vi "Nema GPGGA string to UTM and time.vi"(9 "Grennich Offset":dbl=-8.0, 10 "Antenna offset":dbl max=0.0, 11 "String In (NEAMA GGA)":string="$GPGGA,152703.40,3814.751152,N,12130.720799,W,2,07,1.1,-5.47,M,-23.44,M,3.2,0211\n*5E") -> (0 "date/time string":string, 1 "Elevation":dbl format="%#_8g", 2 "Easting (M)":dbl format="%#.10g", 3 "Northing (M)":dbl format="%#.10g", 4 "Zone (string)":string)   [LabVIEW 2011]
uses:
  <vilib>/Utility/miscctls.llb/LVDateTimeRec.ctl
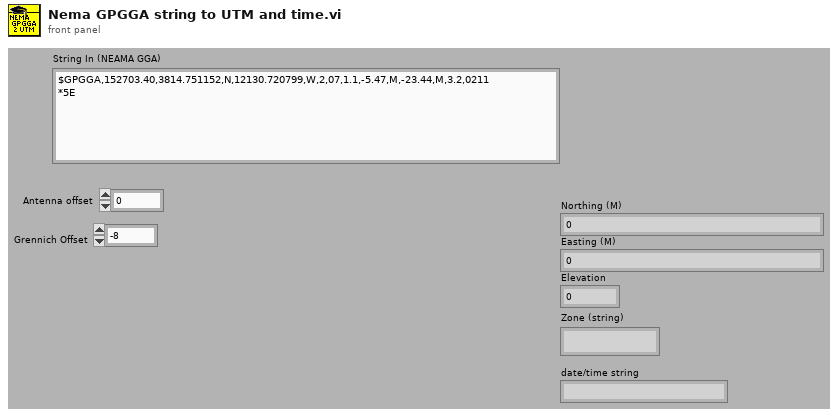
[diagram p1: front panel]
types:
  T1 = typedef "LVDateTimeRec.ctl" = cluster{"fractional second":dbl, "second":i32, "minute":i32, "hour":i32, "day of month":i32, "month":i32, "year":i32, "day of week":i32, "day of year":i32, "DST":i32}
  T2 = cluster{"Time of NEMA":cluster{"Seconds":i32, "Minutes":i32, "Hours":i32}, "Lat-Long in Decimal Degrees":cluster{"Latitude (DD)":dbl, "Longitude (DD)":dbl}, "Point quality variables":cluster{"HDOP":dbl, "#Sats":dbl, "fixQuality":dbl}, "Elevations":cluster{"Elevation (Mean Sea Level)":dbl, "geodal separation":dbl, "Elevation (Height above Elipsode)":dbl}}
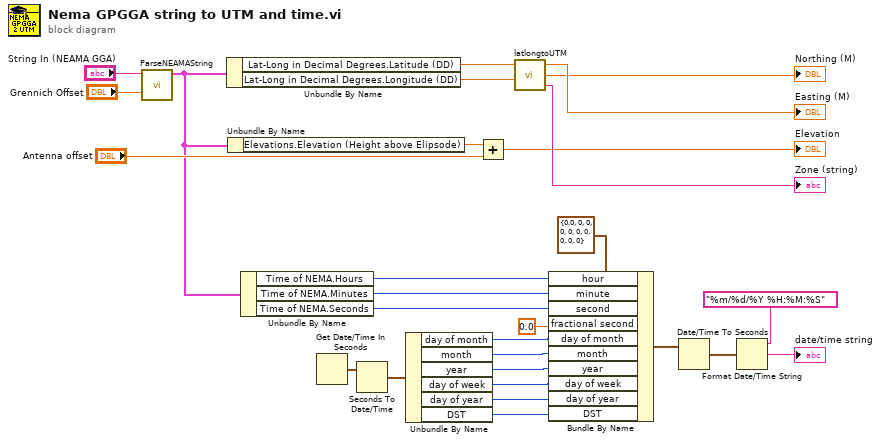
[diagram p0: block diagram]
diagram:
  n1 = call "ParseNEAMAString.vi"("Grennich Offset"="Grennich Offset", "String In (NEAMA GGA)"="String In (NEAMA GGA)") -> ("NEMA string capture variables Out"=w1:T2)  [unwired: 6 in, 1 out]
  n2 = Unbundle By Name(w1) -> ("Lat-Long in Decimal Degrees.Latitude (DD)"=w10:dbl, "Lat-Long in Decimal Degrees.Longitude (DD)"=w9:dbl)
  n3 = Unbundle By Name(w1) -> ("Elevations.Elevation (Height above Elipsode)"=w5:dbl)
  n4 = Unbundle By Name(w1) -> ("Time of NEMA.Hours"=w8:i32, "Time of NEMA.Minutes"=w7:i32, "Time of NEMA.Seconds"=w6:i32)
  n5 = Get Date/Time In Seconds() -> (seconds since 1Jan1904=w24:timestamp)
  n6 = Seconds To Date/Time(time stamp (now)=w24) -> (date time rec=w23:T1)  [unwired: 1 in]
  n7 = Unbundle By Name(w23) -> ("day of month"=w17:i32, "month"=w18:i32, "year"=w19:i32, "day of week"=w20:i32, "day of year"=w21:i32, "DST"=w22:i32)
  n8 = Add(x=w5, y="Antenna offset") -> (x+y=→"Elevation":dbl)
  n9 = call "latlongtoUTM.vi"("Longitude (DD)"=w9, "Latitude (DD)"=w10) -> ("Zone (string)"=→"Zone (string)":string, "Northing (M)"=→"Northing (M)":dbl, "Easting (M)"=→"Easting (M)":dbl)  [unwired: 2 in]
  n10 = Bundle By Name(cluster=T1 {"fractional second"=0.0, "second"=0, "minute"=0, "hour"=0, "day of month"=0, "month"=0, "year"=0, "day of week"=0, "day of year"=0, "DST"=0} ("date time rec"), "hour"=w8, "minute"=w7, "second"=w6, "fractional second"=0.0, "day of month"=w17, "month"=w18, "year"=w19, "day of week"=w20, "day of year"=w21, "DST"=w22) -> (w15:T1)
  n11 = Date/Time To Seconds(2:w15) -> (0:w14:timestamp)  [unwired: 1 in]
  n12 = Format Date/Time String(time format string (%c)="%m/%d/%Y %H:%M:%S", seconds (now)=w14) -> (date/time string=→"date/time string":string)  [unwired: 1 in]
